vi "gxml_QuickParser.vi"(8 "error in (no error)":errorcluster, 9 "TypeDesc":variant, 10 "XML File String":string) -> (0 "error out":errorcluster, 2 "Parsed Data":variant)   [LabVIEW 2011, in "Third Party VIs.lvlib" / "GXML.lvlib"]
doc: "Using a custom XML schema, this VI converts an XML string into a user specified LabVIEW data type. The data structure is defined by the input <b>TypeDesc</b> and its elements must have the same name and hierarchy as the elements in the XML string.\n\nThis VI shoud be used only if you are certain that the specified type definition <b>exactly matches</b> the data type used to create the XML string. The limitation exists because the VI uses no recursion, it simply iterates through the XML string line by line and flattens any data into a binary array. This VI is much faster than its recursive-searching counterpart; however since it does not use the type definition to parse the XML string, it cannot give complete error information (like mismatched datatypes or incorrect order of elements etc.)."
uses:
  GXML.lvlib
  <vilib>/regexp/Match Regular Expression.xnode
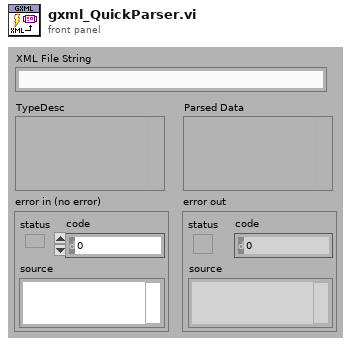
[diagram p1: front panel]
types:
  T1 = cluster{"Hierarchy":string, "Item Name":string, "Empty Array?":bool}
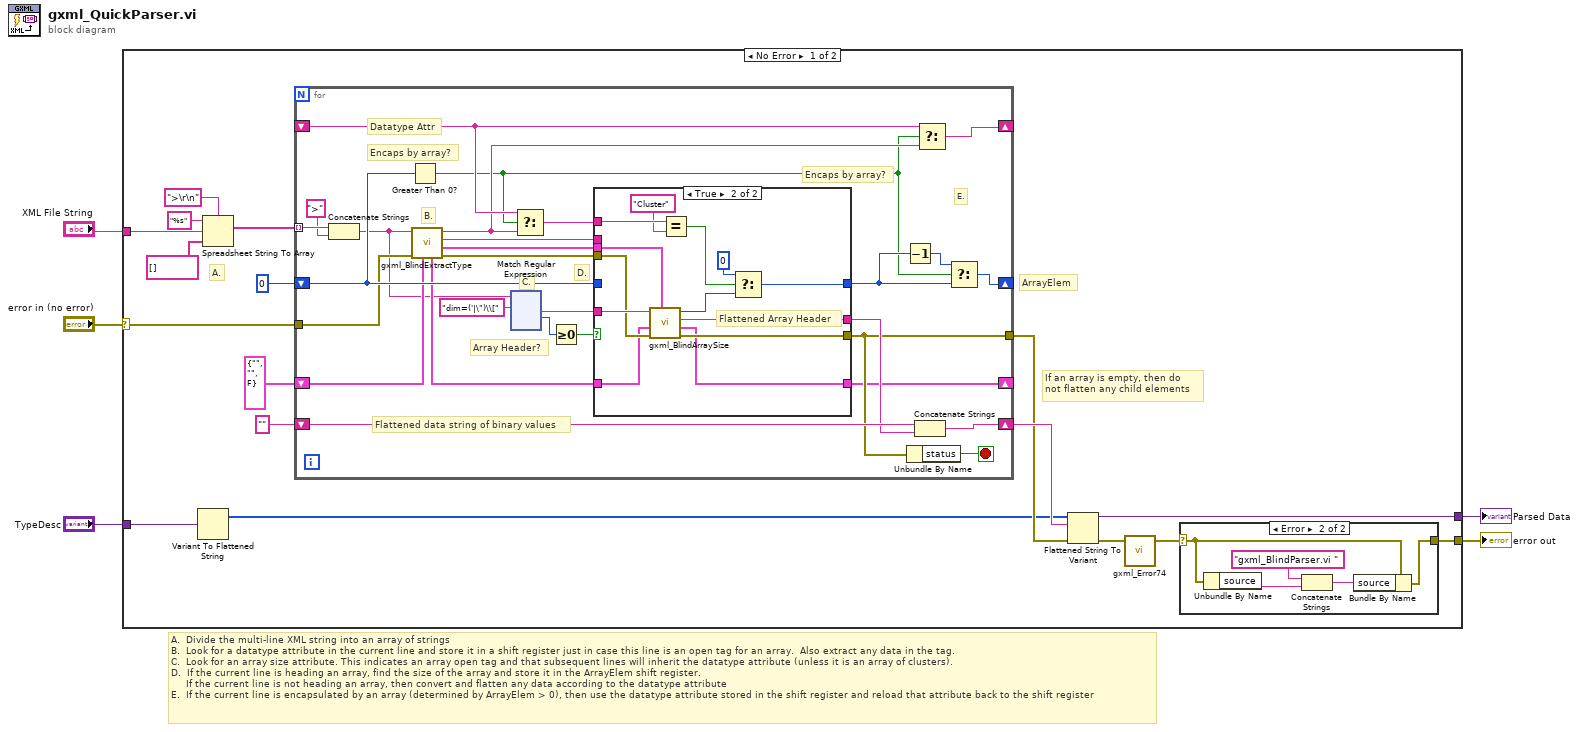
[diagram p0: block diagram]
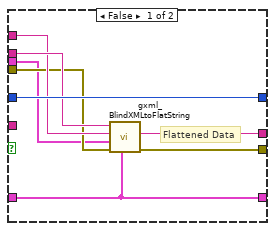
[diagram p3: hidden frame]
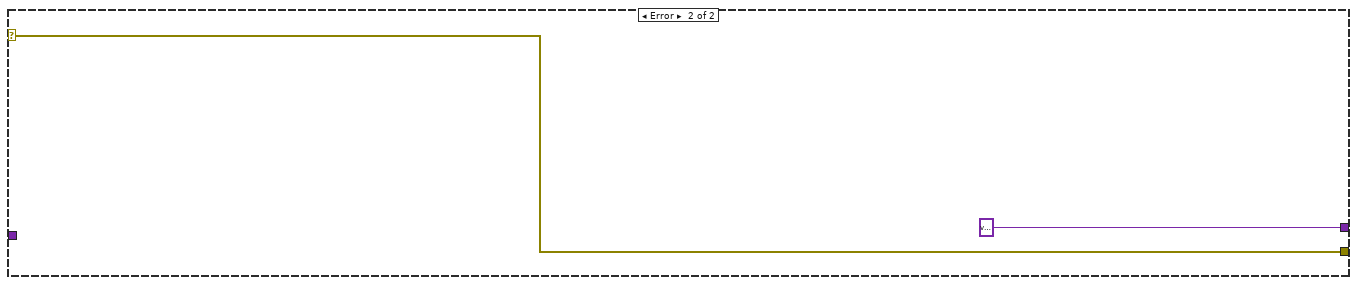
[diagram p4: hidden frame]
diagram:
  # "A.  Divide the multi-line XML string into an array of strings\nB.  Look for a datatype attribute in the current line and store it in a shift register just in case this line is an open tag for an array.  Also extract any data in the tag.\nC.  Look for an array size attribute. This indicates an array open tag and that subsequent lines will inherit the datatype attribute (unless it is an array of clusters).\nD.  If the current line is heading an array, find the size of the array and store it in the ArrayElem shift register.\n     If the current line is not heading an array, then convert and flatten any data according to the datatype attribute\nE.  If the current line is encapsulated by an array (determined by ArrayElem > 0), then use the datatype attribute stored in the shift register and reload that attribute back to the shift register"
  n1 = case shown="No Error" "error in (no error)" {
    selector: "error in (no error)" -> [w12 w189]
    tunnel: "XML File String" -> [w20 _]
    tunnel: [w11 w189] -> w4
    tunnel: [w14 variant ("Variant")] -> w3
    tunnel: "TypeDesc" -> [w13 _]
    frame No Error {
      # "If an array is empty, then do \nnot flatten any child elements"
      # "ArrayElem"
      # "A."
      n2 = Variant To Flattened String(Variant=w13) -> (1:w15:i16[])  [unwired: 1 out]
      n3 = Spreadsheet String To Array(delimiter (Tab)=">\r\n", format string="%s", spreadsheet string=w20, array type (2D Dbl)=string[] []) -> (array=w6:string[])
      n4 = for {
        tunnel: w6 -> [w33] mode=indexing
        shift-right: [w53] -> _
        shift-left: 0 -> [w51]
        shift-right: [w52] -> _
        shift-left: _ -> [w48]
        shift-right: [w43] -> w17
        shift-left: "" -> [w45]
        tunnel: [w42] -> w16
        tunnel: w12 -> [w40]
        shift-right: [w36] -> _
        shift-left: T1 {"Hierarchy"="", "Item Name"="", "Empty Array?"=FALSE} ("Encaps Array Info") -> [w35]
        stop <- w41 stop-if-true
        # "Flattened data string of binary values"
        # "Array Header?"
        # "E."
        # "Encaps by array?"
        # "Encaps by array?"
        # "Datatype Attr"
        # "D."
        # "C."
        # "B."
        n5 = Concatenate Strings(w33, ">") -> (w30:string)
        n6 = Greater Than 0?(x=w51) -> (x > 0?=w46:bool)
        n7 = call "gxml_BlindExtractType.vi"("Encaps Array Info"=w35, "error in"=w40, "XML Line"=w30) -> ("error out"=w38:errorcluster, "Item Name"=w37:cluster{"Hierarchy":string, "Item Name":string}, "Extracted Content"=w39:string, "Extracted Type"=w47:string, "Encaps Array Info Out"=w34:T1)  [unwired: 4 in]
        n8 = xnode "Match Regular Expression"("input string"=w30, "regular expression"="dim=('|\")\\[") -> ("after match"=w54:string, "offset past match"=w29:i32)  [unwired: 4 in, 3 out]
        n9 = Select(t=w48, s=w46, f=w47) -> (s? t:f=w31:string)
        n10 = Greater Or Equal To 0?(x=w29) -> (x >= 0?=w55:bool)
        n11 = case shown="True" w55 {
          tunnel: w31 -> [w173 w187]
          tunnel: w51 -> [w175 _]
          tunnel: w54 -> [_ w188]
          tunnel: [w175 w183] -> w49
          tunnel: w39 -> [w174 _]
          tunnel: [w170 w182] -> w44
          tunnel: [w172 w181] -> w42
          tunnel: w38 -> [w171 w180]
          tunnel: w37 -> [w169 w178]
          tunnel: [w168 w177] -> w36
          tunnel: w34 -> [w168 w176]
          frame False {
            # "Flattened Data"
            n12 = call "gxml_BlindXMLtoFlatString.vi"("Encaps Array Info"=w168, "error in"=w171, "Item Name"=w169, "Datatype"=w173, "Item Contents"=w174) -> ("error out"=w172:errorcluster, "XML Data (Flat Str)"=w170:string)  [unwired: 5 in]
          }
          frame True {
            # "Flattened Array Header"
            n13 = call "gxml_BlindArraySize.vi"("Current Array Info"=w178, "error in"=w180, "Encaps Array Info"=w176, "Dim Attr"=w188) -> ("error out"=w181:errorcluster, "Encaps Array Info"=w177:T1, "Flattened Array Header"=w182:string, "Number of Elements"=w179:i32)  [unwired: 4 in]
            n14 = Equal?(x=w187, y="Cluster") -> (x = y?=w185:bool)
            n15 = Select(t=0, s=w185, f=w179) -> (s? t:f=w183:i32)
          }
        }
        n16 = Decrement(x=w49) -> (x-1=w50:i32)
        n17 = Unbundle By Name(w42) -> ("status"=w41:bool)
        n18 = Concatenate Strings(w45, w44) -> (w43:string)
        n19 = Select(t=w48, s=w46, f=w47) -> (s? t:f=w52:string)
        n20 = Select(t=w50, s=w46, f=w49) -> (s? t:f=w53:i32)
      }
      n21 = Flattened String To Variant(4:w16, 6:w17, 7:w15) -> (0:w10:errorcluster, 3:w14:variant)
      n22 = call "gxml_Error74.vi"("error in (no error)"=w10) -> ("error out"=w9:errorcluster)  [unwired: 4 in]
      n23 = case shown="Error" w9 {
        selector: w9 -> [w23 w26]
        tunnel: [w23 w27] -> w11
        frame No Error {
        }
        frame Error {
          n24 = Unbundle By Name(w26) -> ("source"=w25:string)
          n25 = Concatenate Strings("gxml_BlindParser.vi ", w25) -> (w28:string)
          n26 = Bundle By Name(cluster=w26, "source"=w28) -> (w27:errorcluster)
        }
      }
    }
    frame Error {
    }
  }
  "error out" <- w4
  "Parsed Data" <- w3
